vi "uTTA_GetTimingSettings.vi"(8 "error in":errorcluster, 11 "VISA Refnum in":refnum<visa-resource-name>) -> (0 "error out":errorcluster, 1 "Heating Time":u32, 3 "VISA Refnum out":refnum<visa-resource-name>, 4 "Cooling Time":u32, 5 "PreHeating Time":u32, 7 "Received":string)   [LabVIEW 2021]
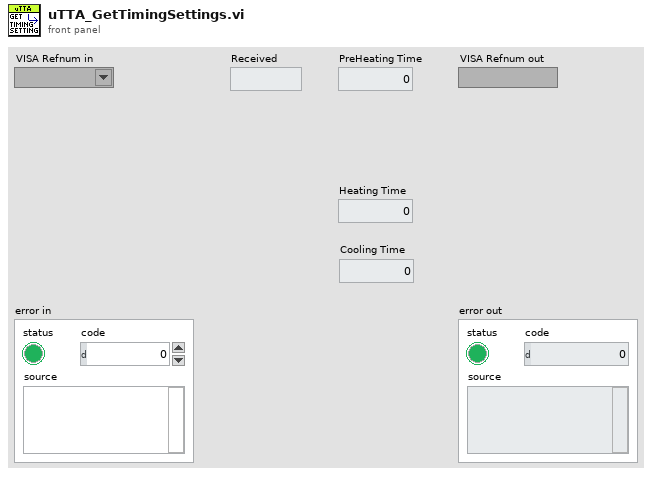
[diagram p1: front panel]
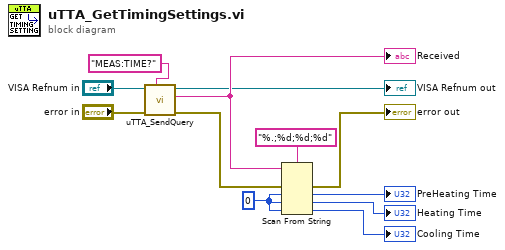
[diagram p0: block diagram]
diagram:
  w3 = u32 0 ("default value 1")
  n1 = call "uTTA_SendQuery.vi"("Send String"="MEAS:TIME?" ("format string"), "error in (no error)"="error in", "VISA Refnum in"="VISA Refnum in") -> ("error out"=w8:errorcluster, "Received"=w6:string, "VISA Refnum out"=→"VISA Refnum out":refnum<visa-resource-name>)  [unwired: 6 in]
  "Received" <- w6
  n2 = Scan From String(format string="%.;%d;%d;%d", input string=w6, error in=w8, default 1=w3, default 2=w3, default 3=w3) -> (error out=→"error out":errorcluster, output 1=→"PreHeating Time":u32, output 2=→"Heating Time":u32, output 3=→"Cooling Time":u32)  [unwired: 1 in, 2 out]
